vi "SwerveAngle.vi"() -> ()   [LabVIEW 2019]
uses:
  <vilib>/Rock Robotics/WPI/ThirdParty/Phoenix-LabVIEW/Motor Controller/Get/CTRE_Phoenix_MotorController_IntegratedSensorData_TalonFX.vi
  <vilib>/Rock Robotics/WPI/ThirdParty/Phoenix-LabVIEW/Motor Controller/Controls/CTRE_Phoenix_MotorControl_ControlMode.ctl
panel:
  in  "wantedAngle":dbl
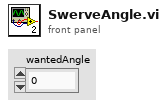
[diagram p1: front panel]
types:
  T1 = typedef "WPI_MotorControlDeviceRef.ctl" = cluster{"DeviceStatus":errorcluster, "Type":T2, "PWM":cluster{"PWM Channel":T3, "DeadBand":T4}, "CAN":cluster{"Device Number":u8, "SetOutput VI Ref":variant, "GetOutput VI Ref":variant, "Enable VI Ref":variant, "Disable VI Ref":variant, "Data":variant}, "Invert":bool, "DIO PWM":cluster{"PWM \"Enable\" Channel":T3, "DIOChannel":T5, "PWM Rate":dbl}}
  T2 = typedef "WPI_MotorControlType.ctl" = enum16{"PWM", "CAN", "DIO PWM"}
  T3 = typedef "FPGA_DIOPWMChannel.ctl" = enum8{"PWM 0", "PWM 1", "PWM 2", "PWM 3", "PWM 4", "PWM 5", "PWM 6", "PWM 7", "PWM 8", "PWM 9", "PWM MXP 0", "PWM MXP 1", "PWM MXP 2", "PWM MXP 3", "PWM MXP 4", "PWM MXP 5", "PWM MXP 6", "PWM MXP 7", "PWM MXP 8", "PWM MXP 9", "Invalid"}
  T4 = typedef "WPI_PWMDeadband.ctl" = cluster{"Name":string, "maxPositivePwm":i32, "minPositivePwm":i32, "centerPwm":i32, "maxNegativePwm":i32, "minNegativePwm":i32, "angularRange":u16}
  T5 = typedef "FPGA_DIOChannel.ctl" = enum8{"DIO 0", "DIO 1", "DIO 2", "DIO 3", "DIO 4", "DIO 5", "DIO 6", "DIO 7", "DIO 8", "DIO 9", "DIO MXP 0", "DIO MXP 1", "DIO MXP 2", "DIO MXP 3", "DIO MXP 4", "DIO MXP 5", "DIO MXP 6", "DIO MXP 7", "DIO MXP 8", "DIO MXP 9", "DIO MXP 10", "DIO MXP 11", "DIO MXP 12", "DIO MXP 13", "DIO MXP 14", "DIO MXP 15", "SPI Port CS1", "SPI Port CS2", "SPI Port CS3", "SPI Port MISO", "SPI Port MOSI", "Invalid"}
  T6 = typedef "CTRE_Phoenix_MotorControl_ControlMode.ctl" = u16
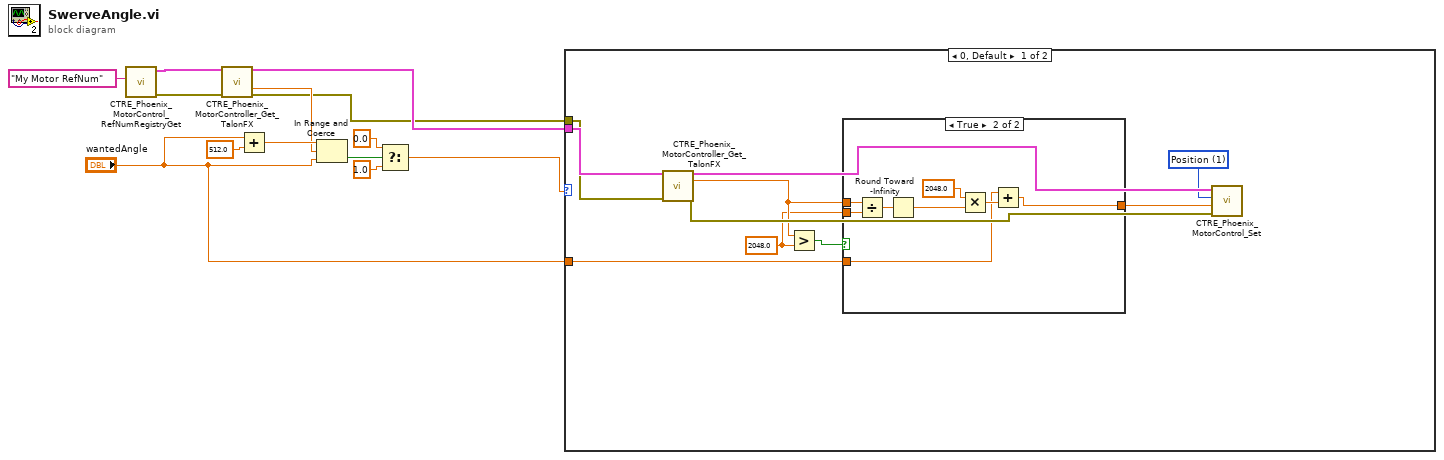
[diagram p0: block diagram]
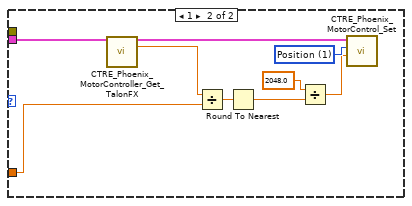
[diagram p3: hidden frame]
diagram:
  n1 = call <vilib>:"CTRE_Phoenix_MotorControl_RefNumRegistryGet.vi"("refnum name"="My Motor RefNum") -> ("error out"=w12:errorcluster, "PhoenixMotorControlDevRef"=w13:T1)  [unwired: 9 in]
  n2 = call-poly <vilib>:"CTRE_Phoenix_MotorController_Get_TalonFX.vi"("PhoenixMotorControlDevRef"=w13, "error in"=w12) -> ("PhoenixMotorControlDevRef"=w9:T1, "Absolute Position"=w4:dbl, "error out"=w2:errorcluster)  [unwired: 9 in, 2 out]
  n3 = Add(x="wantedAngle", y=512.0) -> (x+y=w10:dbl)
  n4 = In Range and Coerce(upper limit=w10, x=w4, lower limit="wantedAngle") -> (In Range?=w8:bool)  [unwired: 1 out]
  n5 = Select(t=0.0, s=w8, f=1.0) -> (s? t:f=w5:dbl)
  n6 = case shown="0, Default" w5 {
    tunnel: w9 -> [w23 w40]
    tunnel: w2 -> [w20 _]
    tunnel: "wantedAngle" -> [w18 w33]
    frame 0, Default {
      w16 = T6 1 items=["PercentOutput"=0, "Position"=1, "Velocity"=2, "Current"=3, "Follower"=5, "MotionProfile"=6, "MotionMagic"=7, "MotionProfileArc"=10, "Disabled"=15] ("Control Mode")
      w14 = 2048.0 ("y")
      n7 = call-poly <vilib>:"CTRE_Phoenix_MotorController_Get_TalonFX.vi"("PhoenixMotorControlDevRef"=w23, "error in"=w20) -> ("PhoenixMotorControlDevRef"=w22:T1, "Position"=w17:dbl, "error out"=w21:errorcluster)  [unwired: 9 in, 2 out]
      n8 = Greater?(x=w17, y=w14) -> (0:w15:bool)
      n9 = case shown="True" w15 {
        tunnel: w17 -> [_ w32]
        tunnel: [w24 w27] -> w19
        tunnel: w18 -> [w24 w26]
        tunnel: w14 -> [_ w25]
        frame False {
        }
        frame True {
          n10 = Divide(x=w32, y=w25) -> (x/y=w31:dbl)
          n11 = Round Toward -Infinity(1:w31) -> (0:w30:dbl)
          n12 = Multiply(x=2048.0, y=w30) -> (x*y=w28:dbl)
          n13 = Add(x=w26, y=w28) -> (x+y=w27:dbl)
        }
      }
      n14 = call <vilib>:"CTRE_Phoenix_MotorControl_Set.vi"("error in (no error)"=w21, "Output"=w19, "Control Mode"=w16, "PhoenixMotorControlDevRef"=w22) -> ()  [unwired: 6 in, 2 out]
    }
    frame 1 {
      w41 = T6 1 items=["PercentOutput"=0, "Position"=1, "Velocity"=2, "Current"=3, "Follower"=5, "MotionProfile"=6, "MotionMagic"=7, "MotionProfileArc"=10, "Disabled"=15] ("Control Mode")
      n15 = call-poly <vilib>:"CTRE_Phoenix_MotorController_Get_TalonFX.vi"("PhoenixMotorControlDevRef"=w40) -> ("PhoenixMotorControlDevRef"=w34:T1, "Position"=w39:dbl)  [unwired: 10 in, 3 out]
      n16 = Divide(x=w39, y=w33) -> (x/y=w38:dbl)
      n17 = Round To Nearest(number=w38) -> (nearest integer value=w37:dbl)
      n18 = Divide(x=2048.0, y=w37) -> (x/y=w35:dbl)
      n19 = call <vilib>:"CTRE_Phoenix_MotorControl_Set.vi"("Output"=w35, "Control Mode"=w41, "PhoenixMotorControlDevRef"=w34) -> ()  [unwired: 7 in, 2 out]
    }
  }
